vi "Init Keyboard.vi"   [LabVIEW 2018]
uses:
  Global Teleop Variables.vi
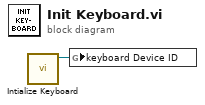
[diagram p0: block diagram]
diagram:
  n1 = call <vilib>:"Intialize Keyboard.vi"() -> ("device ID"=w1:refnum<k1>)  [unwired: 10 in, 1 out]
  n2 = global write "Global Teleop Variables.vi" "keyboard Device ID"(w1) -> ()
